vi "Cleanup.vi"(8 "error in (no error)":errorcluster, 11 "Panel in":refnum<class "Panel.lvclass">) -> (0 "error out":errorcluster)   [LabVIEW 2020, in "OOPanel.lvlib" / "Panel.lvclass"]
uses:
  Panel.lvclass
  Panel.lvclass/Panel.ctl
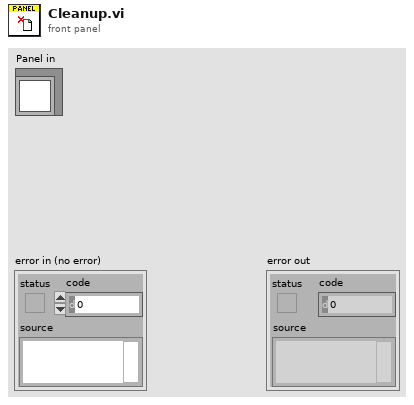
[diagram p1: front panel]
types:
  T1 = typedef "OOPanel.lvlib/Panel.lvclass/Ref Data.ctl" = cluster{"Panel Ref":refnum<vi>, "SubPanel":refnum<vi>, "Close":bool, "Running":bool, "State":T2}
  T2 = typedef "OOPanel.lvlib/Panel.lvclass/Visibility State.ctl" = enum16{"Idle", "Closed", "Hidden", "Visible", "Subpanel"}
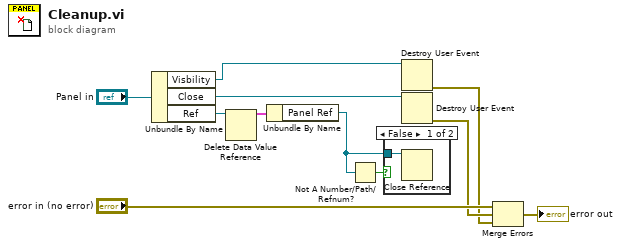
[diagram p0: block diagram]
diagram:
  n1 = Unbundle By Name("Panel in") -> ("Visbility"=w1:refnum<user-event>, "Close"=w2:refnum<user-event>, "Ref"=w10:refnum<data-value>)
  n2 = Delete Data Value Reference(data value reference=w10) -> (data value=w9:T1)  [unwired: 1 in, 1 out]
  n3 = Unbundle By Name(w9) -> ("Panel Ref"=w8:refnum<vi>)
  n4 = Not A Number/Path/Refnum?(number/path/refnum=w8) -> (NaN/Path/Refnum?=w7:bool)
  n5 = case shown="False" w7 {
    tunnel: w8 -> [w12 _]
    frame False {
      n6 = Close Reference(reference=w12) -> ()  [unwired: 1 in, 1 out]
    }
    frame True {
    }
  }
  n7 = Destroy User Event(user event=w1) -> (error out=w4:errorcluster)  [unwired: 1 in]
  n8 = Destroy User Event(user event=w2) -> (error out=w5:errorcluster)  [unwired: 1 in]
  n9 = Merge Errors("error in (no error)", w5, w4) -> (→"error out":errorcluster)
